vi "Amp_PS_set.vi"(0 "delay before read (ms)":u32=500, 1 "Set Control":string(combo), 2 "Set Value":dbl min=0.0 max=30.0 step=0.1, 3 "error in (no error)":errorcluster, 4 "Amp PS address":refnum<visa-resource-name>) -> (5 "status":bool, 6 "output cluster":T1)   [LabVIEW 2010]
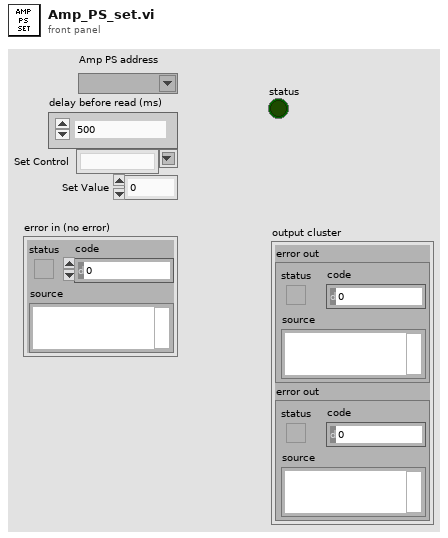
[diagram p1: front panel]
types:
  T1 = cluster{"error out":errorcluster, "error out":errorcluster}
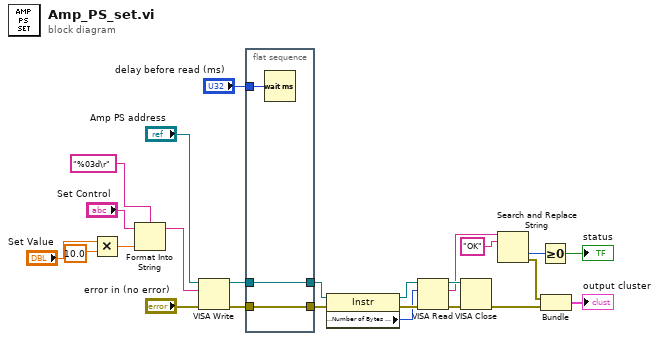
[diagram p0: block diagram]
diagram:
  n1 = Multiply(x="Set Value", y=10.0) -> (x*y=w8:dbl)
  n2 = Format Into String(format string="%03d\r", initial string="Set Control", w8) -> (resulting string=w5:string)  [unwired: 1 in, 1 out]
  n3 = VISA Write(VISA resource name="Amp PS address", write buffer=w5, error in (no error)="error in (no error)") -> (VISA resource name out=w21:refnum<visa-resource-name>, error out=w23:errorcluster)  [unwired: 1 out]
  n4 = flat-sequence {
    tunnel: w23 -> [w27]
    tunnel: [w27] -> w22
    tunnel: w21 -> [w26]
    tunnel: [w26] -> w20
    tunnel: "delay before read (ms)" -> [w28]
    frame #0 {
      n5 = Wait (ms)(milliseconds to wait=w28) -> ()  [unwired: 1 out]
    }
  }
  n6 = property class="Instr"(reference=w20, error in=w22) -> (reference out=w19:refnum<visa-resource-name>, error out=w18:errorcluster, "Serial Settings:Number of Bytes at Serial Port"=w17:u32)
  n7 = VISA Read(VISA resource name=w19, byte count=w17, error in (no error)=w18) -> (VISA resource name out=w24:refnum<visa-resource-name>, read buffer=w13:string, error out=w25:errorcluster)  [unwired: 1 out]
  n8 = VISA Close(VISA resource name=w24, error in (no error)=w25) -> (error out=w2:errorcluster)
  n9 = Search and Replace String(input string=w13, search string="OK" ("true string")) -> (offset past replacement=w11:i32, error out=w3:errorcluster)  [unwired: 6 in, 2 out]
  n10 = Greater Or Equal To 0?(x=w11) -> (x >= 0?=→"status":bool)
  n11 = Bundle("error out"=w3, "error out"=w2) -> (→"output cluster":T1)  [unwired: 1 in]
